vi "Main.vi"() -> ()   [LabVIEW 2026]
doc: "============================================================\nPI-C867-IO Control — VI Principal\nVersion : 0.0\nDate : Avril 2026\nAuteur : Institut Fresnel / Photonics Platform\n============================================================\n\nDESCRIPTION\n-----------\nVI de pilotage multi-positions du contrôleur PI C-867 pour\nmicroscopie de polarisation. Gère la séquence de déplacement\nXY synchronisée avec l'acquisition (lasers, polariseurs, caméra)\nvia signaux TTL hardware sans dialogue RS-232 pendant la DAQ.\n\nFACE AVANT\n----------\nEntrées :\n - Tableau XY (Nx2 DBL) : positions en mm\n - Nb boucles (I32) : nombre de répétitions de la séquence\n - Bouton Go : démarre la séquence\n - Bouton Stop : arrêt immédiat\n\nIndicateurs :\n - Position courante : ex. \"3 / 5\"\n - Boucle courante : ex. \"2 / 3\"\n - État : message texte (Initialisé / En cours / Arrêté)\n - Erreur : code et description\n\nMACHINE À ÉTATS\n---------------\nINIT ? Connexion C-867 (USB), SVO, FRF\n Init task CO (GO) et task DI (READY)\nWAIT_FOR_EVENT ? Attente bouton Go ou Quitter\nLOAD_POSITIONS ? Envoi macro via Python (main.py)\nRUNNING ? Émission impulsion GO (compteur CO)\nWAIT_READY ? Attente front montant READY (Change Detection)\nACQUIRE ? Acquisition (1s en test) + gestion boucles\nSTOP ? Arrêt C-867, clear tasks DAQ\n\nCONNEXIONS HARDWARE\n-------------------\nC-867 broche 4 (jaune) ? PFI13 Dev USB-6353-3 (GO)\nC-867 broche 5 (violet) ? P0.4 Dev USB-6353-3 (READY)\nGND (blindage) ? DGND\n\nDÉPENDANCES\n-----------\n- PI GCS LabVIEW VIs (C:\\ProgramData\\PI\\LabVIEW\\)\n- Python 3.x + PIPython\n- Scripts : main.py, macro_builder.py\n- NI-DAQmx\n============================================================"
uses:
  SubVI/Controls/Etats.ctl
  SubVI/Controls/TypeDef_FGV.ctl
  <vilib>/DAQmx/read.llb/DAQmx Read (Digital Bool 1Line 1Point).vi
  <vilib>/DAQmx/miscellaneous.llb/DAQmx Fill In Error Info.vi
panel:
  out "Current loop":u32=1
  out "Current pos":i32=1
  in  "Emergency stop":bool
  in  "# of Loops":dbl=3.0
  in  "Position table":dbl[][](array[numeric])=[[0.0, 0.0, 0.0], [0.1, 0.1, 0.0], [0.2, 0.2, 0.0], [0.3, 0.3, 0.0], [0.1, 0.2, 0.0]]
  out "error out":errorcluster caption="sortie d'erreur"
  in  "error in":errorcluster caption="entrée d'erreur"
  in  "Arrêter":bool
  in  "GO":bool
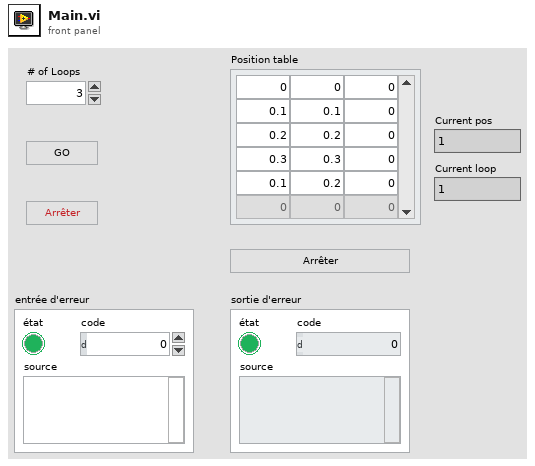
[diagram p1: front panel]
types:
  T1 = typedef "TypeDef_FGV.ctl" = enum16{"Initialize", "Write", "Read"}
  T2 = typedef "Etats.ctl" = enum16{"INIT", "WAIT_FOR_EVENT", "LOAD_POSITIONS", "RUNNING", "WAIT_READY", "ACQUIRE", "STOP"}
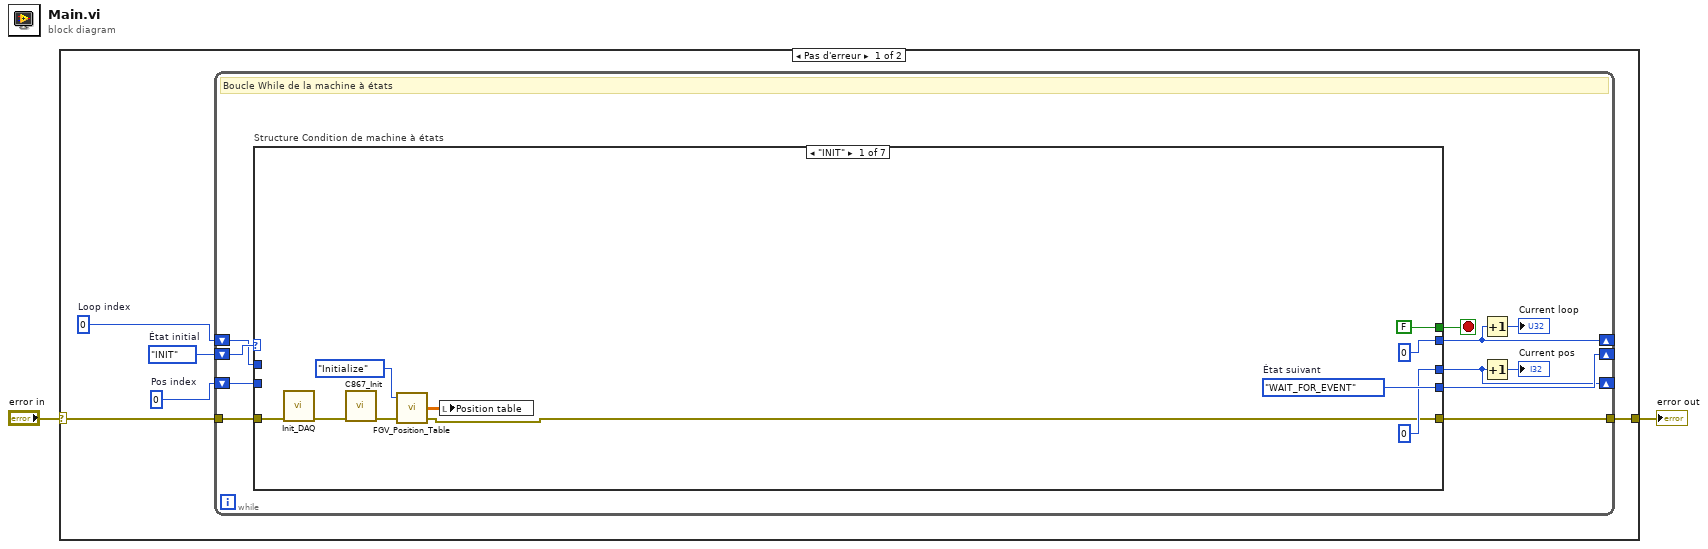
[diagram p0: block diagram]
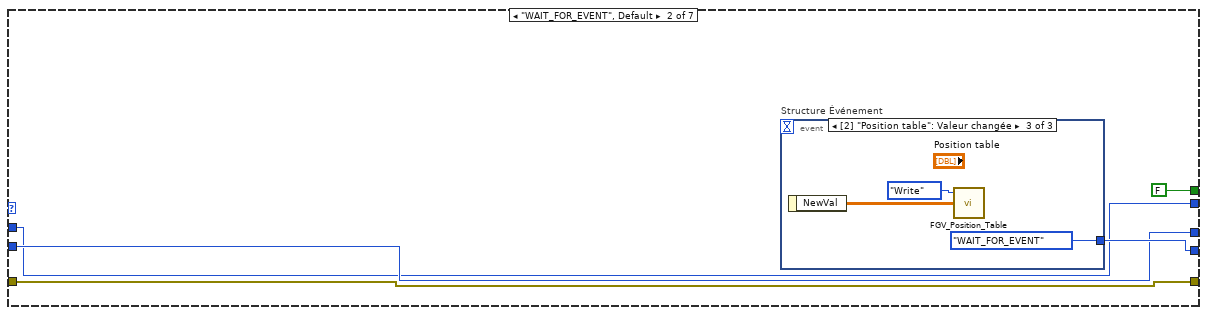
[diagram p2: hidden frame]
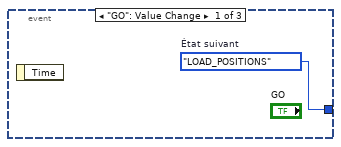
[diagram p3: hidden frame]
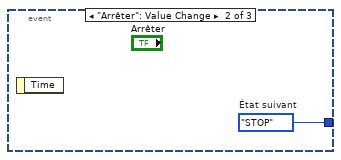
[diagram p4: hidden frame]
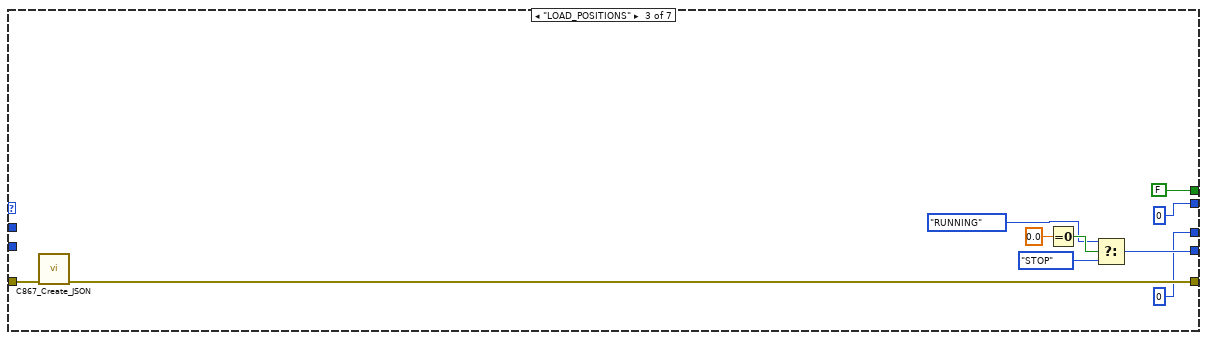
[diagram p5: hidden frame]
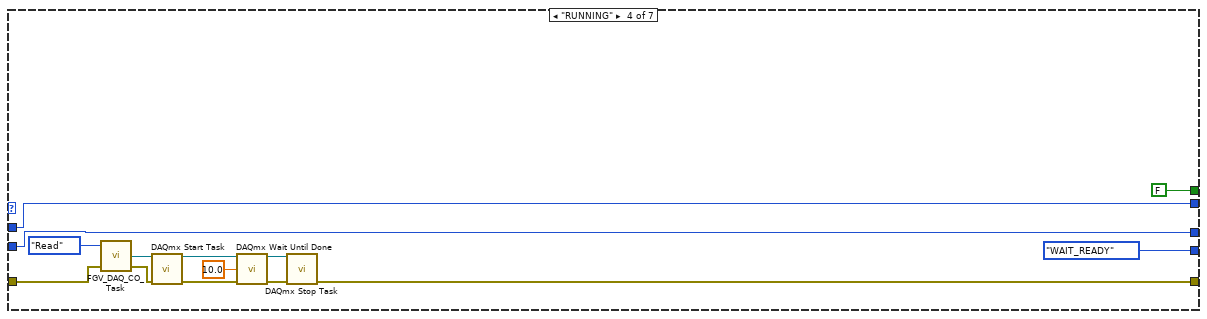
[diagram p6: hidden frame]
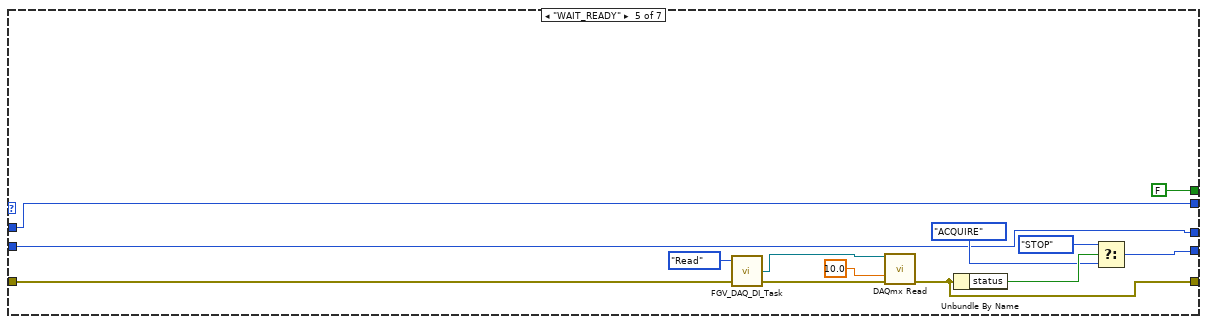
[diagram p7: hidden frame]
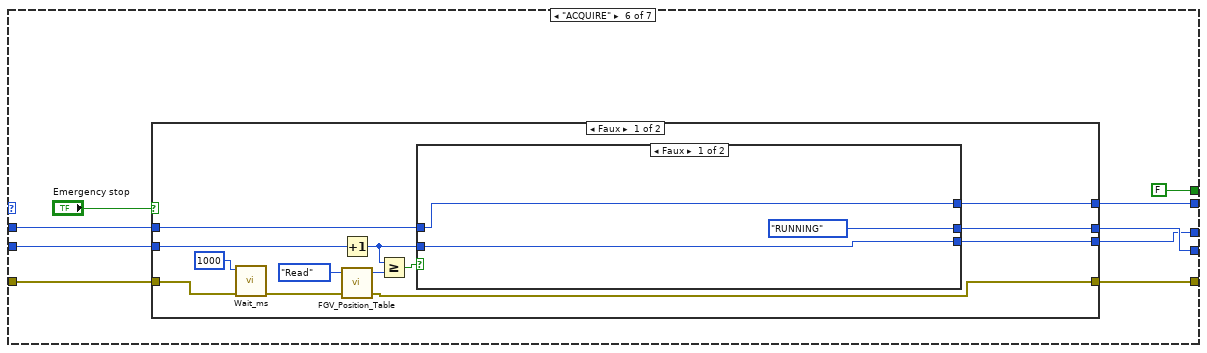
[diagram p8: hidden frame]
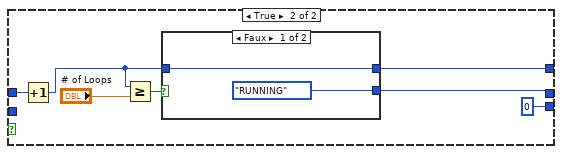
[diagram p9: hidden frame]
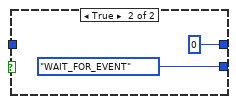
[diagram p10: hidden frame]
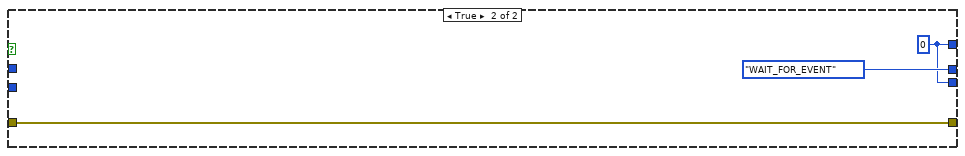
[diagram p11: hidden frame]
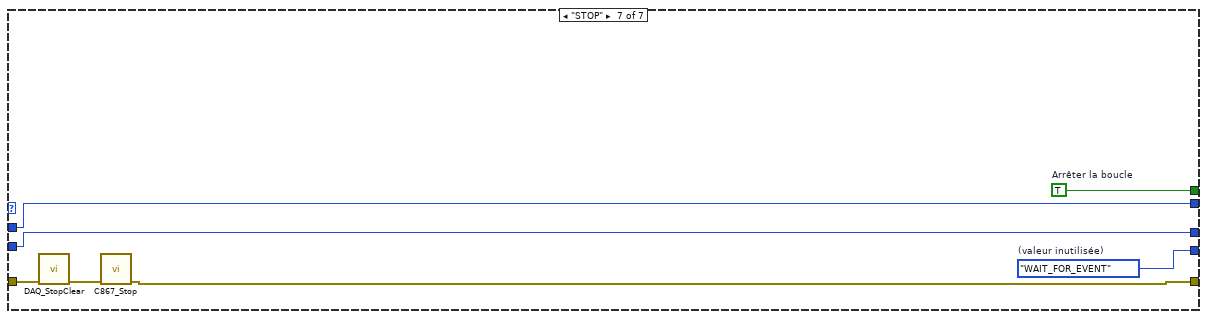
[diagram p12: hidden frame]
diagram:
  n1 = case shown="Pas d'erreur" "error in" {
    selector: "error in" -> [w6 w122]
    tunnel: [w5 w122] -> w1
    frame No Error {
      w3 = 0  # Loop index
      w4 = 0  # Pos index
      w7 = Etats."INIT"  # État initial
      n2 = while {
        shift-right: [w17] -> _
        shift-left: w7 -> [w18]
        tunnel: w6 -> [w15]
        tunnel: [w14] -> w5
        shift-right: [w13] -> _
        shift-left: w4 -> [w11]
        shift-right: [w12] -> _
        shift-left: w3 -> [w10]
        stop <- w16 stop-if-true
        # "Boucle While de la machine à états"
        n3 = case "Structure Condition de machine à états" shown="\"INIT\"" w18 {
          tunnel: [w28 w33 w42 Etats."WAIT_READY" ("(valeur inutilisée)") w67 w80 w121] -> w17
          tunnel: [FALSE ("Arrêter la boucle") FALSE ("Arrêter la boucle") FALSE ("Arrêter la boucle") FALSE ("Arrêter la boucle") FALSE ("Arrêter la boucle") FALSE ("Arrêter la boucle") w120] -> w16
          tunnel: w15 -> [w26 w31 w47 w57 w74 w82 w119]
          tunnel: [w20 w31 w46 w51 w70 w81 w115] -> w14
          tunnel: [0 ("Pos index") w30 0 ("Pos index") w50 w64 w79 w118] -> w13
          tunnel: [u32 0 ("milliseconds to wait") w29 u32 0 ("milliseconds to wait") w49 w63 w78 w117] -> w12
          tunnel: w11 -> [_ w30 _ w50 w64 w77 w118]
          tunnel: w10 -> [_ w29 _ w49 w63 w76 w117]
          frame "INIT" {
            w28 = Etats."WAIT_FOR_EVENT"  # État suivant
            n4 = call "Init_DAQ.vi"("error in"=w26) -> ("error out"=w25:errorcluster)  [unwired: 10 in]
            n5 = call "C867_Init.vi"("error in"=w25) -> ("error out"=w22:errorcluster)  [unwired: 10 in]
            n6 = call "FGV_Position_Table.vi"("error in"=w22, "Action"=TypeDef_FGV."Initialize") -> ("error out"=w20:errorcluster, "Position table"=w19:dbl[][])  [unwired: 1 in, 1 out]
            n7 = local write "Position table"(w19) -> ()
          }
          frame "WAIT_FOR_EVENT", Default {
            n8 = event "Structure Événement" shown="[2] \"Position table\": Valeur changée" {
              selector: _ -> [_ _ _]
              dyn-events: _ -> [_ _ _]
              timeout: _ -> [_ _ _]
              tunnel: [w34 w35 Etats."WAIT_FOR_EVENT" ("État suivant")] -> w33
              event "GO": Value Change {
                w34 = Etats."LOAD_POSITIONS"  # État suivant
                n9 = event-data() -> ()  [unwired: 1 in, 1 out]
              }
              event "Arrêter": Value Change {
                w35 = Etats."STOP"  # État suivant
                n10 = event-data() -> ()  [unwired: 1 in, 1 out]
              }
              event "Position table": Value Change {
                n11 = event-data() -> ("NewVal"=w38:dbl[][])  [unwired: 1 in]
                n12 = call "FGV_Position_Table.vi"("Position table"=w38, "Action"=TypeDef_FGV."Write") -> ()  [unwired: 1 in, 3 out]
              }
            }
          }
          frame "LOAD_POSITIONS" {
            n13 = call "C867_Create_JSON.vi"("error in"=w47) -> ("error out"=w46:errorcluster)  [unwired: 9 in, 1 out]
            n14 = Equal To 0?(x=0.0) -> (x = 0?=w45:bool)
            n15 = Select(t=Etats."RUNNING" ("(valeur inutilisée)"), s=w45, f=Etats."STOP" ("cas faux")) -> (s? t:f=w42:T2)
          }
          frame "RUNNING" {
            n16 = call "FGV_DAQ_CO_Task.vi"("error in"=w57, "Action"=TypeDef_FGV."Read") -> ("error out"=w60:errorcluster, "CO task"=w59:refnum<k21>)  [unwired: 2 in]
            n17 = call <vilib>:"DAQmx Start Task.vi"("task/channels in"=w59, "error in"=w60) -> ("task out"=w56:refnum<k21>, "error out"=w54:errorcluster)  [unwired: 12 in]
            n18 = call <vilib>:"DAQmx Wait Until Done.vi"("task/channels in"=w56, "timeout (sec)"=10.0, "error in"=w54) -> ("task out"=w53:refnum<k21>, "error out"=w52:errorcluster)  [unwired: 11 in]
            n19 = call <vilib>:"DAQmx Stop Task.vi"("task/channels in"=w53, "error in"=w52) -> ("error out"=w51:errorcluster)  [unwired: 12 in, 1 out]
          }
          frame "WAIT_READY" {
            n20 = call "FGV_DAQ_DI_Task.vi"("error in"=w74, "Action"=TypeDef_FGV."Read") -> ("error out"=w73:errorcluster, "DI task"=w72:refnum<k21>)  [unwired: 2 in]
            n21 = call-poly <vilib>:"DAQmx Read.vi"("task/channels in"=w72, "timeout"=10.0, "error in"=w73) -> ("error out"=w70:errorcluster)  [unwired: 10 in, 2 out]
            n22 = Unbundle By Name(w70) -> ("status"=w69:bool)
            n23 = Select(t=Etats."STOP" ("(valeur inutilisée)"), s=w69, f=Etats."ACQUIRE" ("(valeur inutilisée)")) -> (s? t:f=w67:T2)
          }
          frame "ACQUIRE" {
            n24 = case shown="Faux" "Emergency stop" {
              tunnel: w82 -> [w96 w113]
              tunnel: [w92 w113] -> w81
              tunnel: [w90 Etats."WAIT_FOR_EVENT" ("(valeur inutilisée)")] -> w80
              tunnel: [w88 w112] -> w79
              tunnel: [w87 w112] -> w78
              tunnel: w77 -> [w89 _]
              tunnel: w76 -> [w86 _]
              frame False {
                n25 = call "Wait_ms.vi"("error in (no error)"=w96, "milliseconds to wait"=u32 1000) -> ("error out"=w94:errorcluster)  [unwired: 9 in]
                n26 = Increment(x=w89) -> (x+1=w91:i32)
                n27 = call "FGV_Position_Table.vi"("error in"=w94, "Action"=TypeDef_FGV."Read") -> ("error out"=w92:errorcluster, "N pos"=w85:i32)  [unwired: 1 in, 1 out]
                n28 = Greater Or Equal?(x=w91, y=w85) -> (x >= y?=w95:bool)
                n29 = case shown="Faux" w95 {
                  tunnel: w91 -> [w99 _]
                  tunnel: [Etats."RUNNING" ("(valeur inutilisée)") w105] -> w90
                  tunnel: [w99 0] -> w88
                  tunnel: [w98 w102] -> w87
                  tunnel: w86 -> [w98 w101]
                  frame False {
                  }
                  frame True {
                    n30 = Increment(x=w101) -> (x+1=w104:u32)
                    n31 = Greater Or Equal?(x=w104, y="# of Loops") -> (x >= y?=w106:bool)
                    n32 = case shown="Faux" w106 {
                      tunnel: [w108 u32 0 ("milliseconds to wait")] -> w102
                      tunnel: [Etats."RUNNING" ("(valeur inutilisée)") Etats."WAIT_FOR_EVENT" ("(valeur inutilisée)")] -> w105
                      tunnel: w104 -> [w108 _]
                      frame False {
                      }
                      frame True {
                      }
                    }
                  }
                }
              }
              frame True {
                w112 = 0
              }
            }
          }
          frame "STOP" {
            w120 = TRUE  # Arrêter la boucle
            w121 = Etats."WAIT_FOR_EVENT"  # (valeur inutilisée)
            n33 = call "DAQ_StopClear.vi"("error in"=w119) -> ("error out"=w116:errorcluster)  [unwired: 10 in]
            n34 = call "C867_Stop.vi"("error in"=w116) -> ("error out"=w115:errorcluster)  [unwired: 10 in]
          }
        }
        n35 = Increment(x=w12) -> (x+1=→"Current loop":u32)
        n36 = Increment(x=w13) -> (x+1=→"Current pos":i32)
      }
    }
    frame Error {
    }
  }
  "error out" <- w1
